vi "CHROMA Get System Status.vi"(8 "Error In":errorcluster, 11 "CHROMA VISA In":refnum<visa-resource-name>) -> (0 "Error Out":errorcluster, 2 "Chroma Data":string[][](array[string]), 3 "CHROMA VISA Out":refnum<visa-resource-name>)   [LabVIEW 2016]
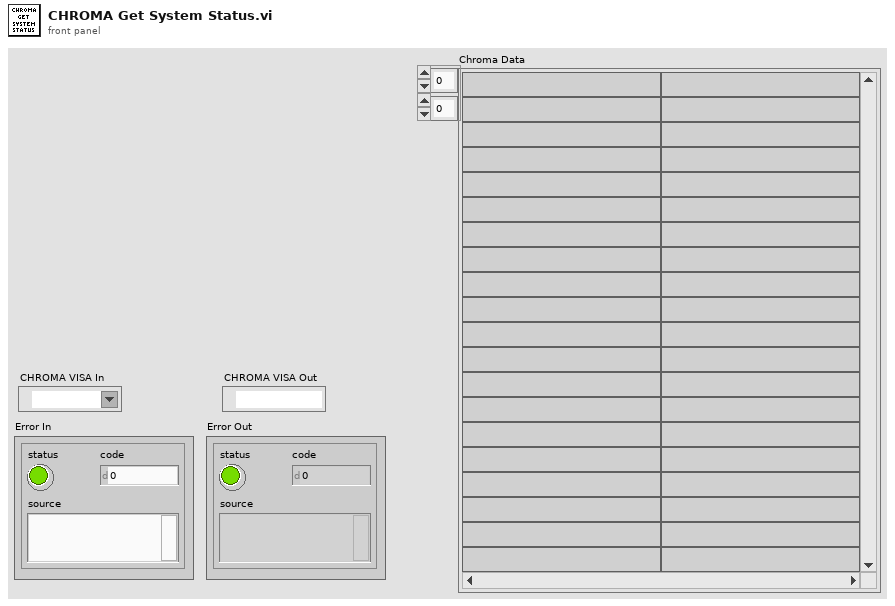
[diagram p1: front panel]
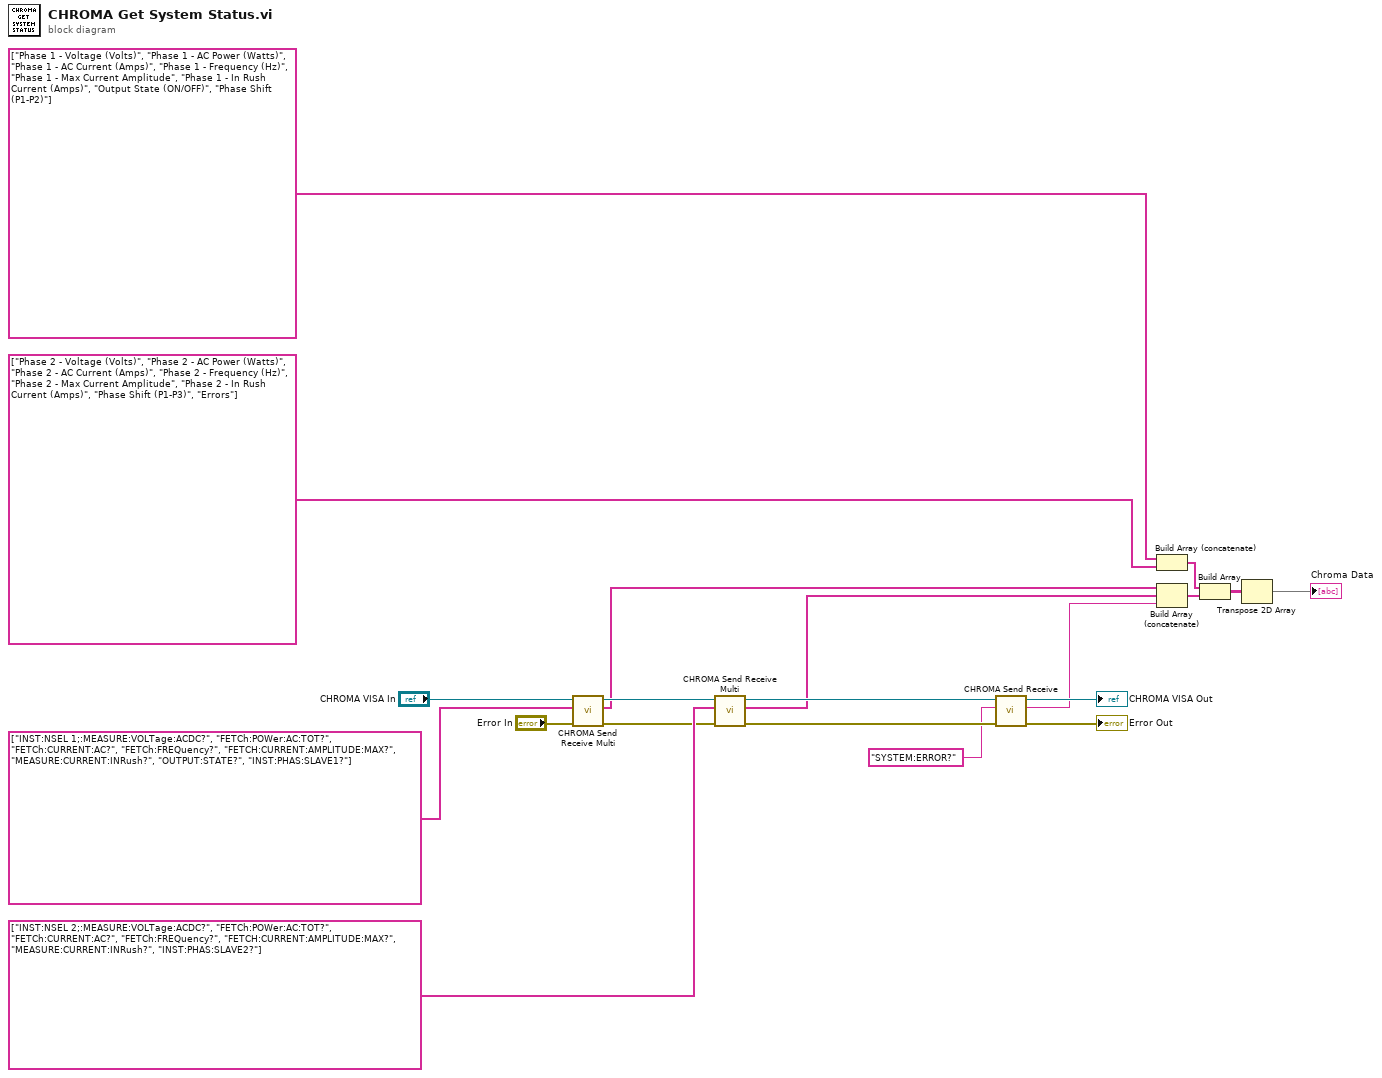
[diagram p0: block diagram]
diagram:
  n1 = call "CHROMA Send Receive Multi.vi"("Error In"="Error In", "Array of Commands"=string[] ["INST:NSEL 1;:MEASURE:VOLTage:ACDC?", "FETCh:POWer:AC:TOT?", "FETCh:CURRENT:AC?", "FETCh:FREQuency?", "FETCH:CURRENT:AMPLITUDE:MAX?", "MEASURE:CURRENT:INRush?", "OUTPUT:STATE?", "INST:PHAS:SLAVE1?"], "CHROMA VISA In"="CHROMA VISA In") -> ("Error Out"=w16:errorcluster, "Array of Results"=w9:string[], "CHROMA VISA Out"=w17:refnum<visa-resource-name>)  [unwired: 6 in]
  n2 = call "CHROMA Send Receive Multi.vi"("Error In"=w16, "Array of Commands"=string[] ["INST:NSEL 2;:MEASURE:VOLTage:ACDC?", "FETCh:POWer:AC:TOT?", "FETCh:CURRENT:AC?", "FETCh:FREQuency?", "FETCH:CURRENT:AMPLITUDE:MAX?", "MEASURE:CURRENT:INRush?", "INST:PHAS:SLAVE2?"], "CHROMA VISA In"=w17) -> ("Error Out"=w14:errorcluster, "Array of Results"=w8:string[], "CHROMA VISA Out"=w11:refnum<visa-resource-name>)  [unwired: 6 in]
  n3 = call "CHROMA Send Receive.vi"("error in (no error)"=w14, "Send Command"="SYSTEM:ERROR?" ("string to write"), "CHROMA VISA In"=w11) -> ("error out"=→"Error Out":errorcluster, "read buffer"=w7:string, "CHROMA VISA Out"=→"CHROMA VISA Out":refnum<visa-resource-name>)  [unwired: 6 in]
  n4 = Build Array (concatenate)(string[] ["Phase 1 - Voltage (Volts)", "Phase 1 - AC Power (Watts)", "Phase 1 - AC Current (Amps)", "Phase 1 - Frequency (Hz)", "Phase 1 - Max Current Amplitude", "Phase 1 - In Rush Current (Amps)", "Output State (ON/OFF)", "Phase Shift (P1-P2)"], string[] ["Phase 2 - Voltage (Volts)", "Phase 2 - AC Power (Watts)", "Phase 2 - AC Current (Amps)", "Phase 2 - Frequency (Hz)", "Phase 2 - Max Current Amplitude", "Phase 2 - In Rush Current (Amps)", "Phase Shift (P1-P3)", "Errors"]) -> (w4:string[])
  n5 = Build Array (concatenate)(w9, w8, w7) -> (w3:string[])
  n6 = Build Array(w4, w3) -> (w2:string[][])
  n7 = Transpose 2D Array(2D array=w2) -> (transposed array=→"Chroma Data":string[][])
